vi "Handle and Broadcast Event.vi"(8 "error in (no error)":errorcluster, 9 "Event Data":refnum<class "Event.lvclass">, 10 "View Enqueuer":refnum<class "Message Enqueuer.lvclass">, 11 "Controller in":refnum<class "Controller.lvclass">) -> (0 "error out":errorcluster, 3 "Controller out":refnum<class "Controller.lvclass">)   [LabVIEW 2023, in "MVC Actors.lvlib" / "Controller.lvclass"]
doc: "This method generates/fires the Event wired to the input triggered by a View. Firing an event originating form a View looks up all actors, but the originating View, who registered to listen to this Event and sends to them this Event on a Zero Coupling based message defined during registration. Errors on broadcasting the event i.e. enqueuer of the registrant not existing, are ignored.\n\n<b>IMPORTANT</b> - Only call this method directly (not through the corresponding message) within actor method calls of your Controller Actor. From helper loops send to self the corresponding message by means of its send method. This is to make sure your controller acts all the currently registered listeners."
uses:
  Controller.lvclass
  <vilib>/ActorFramework/Message Enqueuer/Message Enqueuer.lvclass
  Event/Event.lvclass
  Controller.lvclass/Controller.ctl
  Event Handlers/Abstract Event Message for View/Abstract Event Message for View.lvclass/Abstract Event Message for View.ctl
  <vilib>/ActorFramework/Message Enqueuer/Message Enqueuer.lvclass/Message Enqueuer.ctl
  Event Handlers/Abstract Event Message for View/Send Abstract Event Message for View.vi
  <vilib>/Utility/error.llb/Clear Errors.vi
  <vilib>/ActorFramework/Message Enqueuer/Enqueue.vi
  Event Handlers/Abstract Event Message for View/Abstract Event Message for View.lvclass
  C:/Program Files/National Instruments/LabVIEW 2023/vi.lib/ActorFramework/Message/Message.lvclass
  <vilib>/Utility/LVClass/Get LV Class Name.vi
  <resource>/AFDebug/Generate Trace for Message.vi
  <vilib>/ActorFramework/Message Priority Queue/Priority Enqueue.vi
  Event Handlers/Abstract Event Handler for Controller/Abstract Event Handler for Controller.lvclass
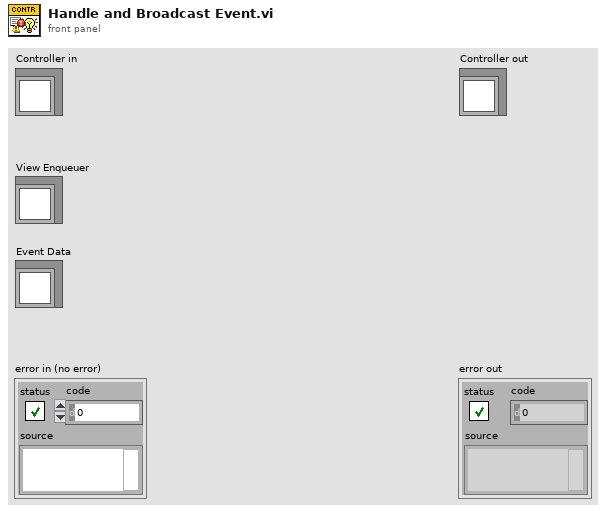
[diagram p1: front panel]
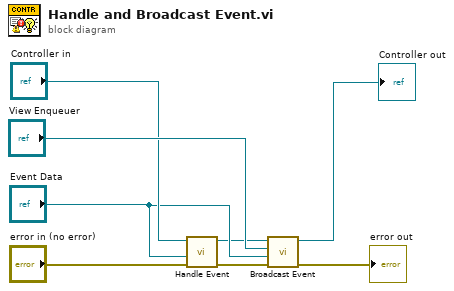
[diagram p0: block diagram]
diagram:
  n1 = call "Handle Event.vi"("error in (no error)"="error in (no error)", "Event Data"="Event Data", "Controller Actor in"="Controller in") -> ("error out"=w1:errorcluster, "Controller Actor out"=w3:refnum<class "Controller.lvclass">)  [unwired: 7 in]
  n2 = call "Broadcast Event.vi"("error in (no error)"=w1, "Event Data"="Event Data", "View Enqueuer"="View Enqueuer", "Controller in"=w3) -> ("error out"=→"error out":errorcluster, "Controller out"=→"Controller out":refnum<class "Controller.lvclass">)  [unwired: 6 in]
